vi "VI Tree.vi"   [LabVIEW 2012, in "Lake Shore Cryotronics 370.lvlib"]
doc: "This is the instrument driver for the LakeShore Cryotronics Model 370 AC Resistance Bridge. The VI Tree displays all the user-callable VIs of the instrument driver in an organized table."
uses:
  <instrlib>/Lake Shore Cryotronics 370/Lake Shore Cryotronics 370.lvlib
panel:
  # "(c) 2001- 2009 National Instruments.  ALL RIGHTS RESERVED."
  # "SEE DIAGRAM\nFOR VI TREE."
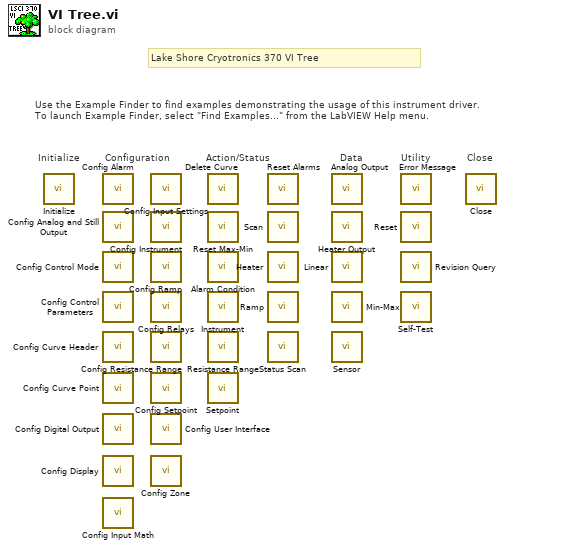
[diagram p0: block diagram]
diagram:
  # "Lake Shore Cryotronics 370 VI Tree"
  # "Initialize"
  # "Close"
  # "Action/Status"
  # "Data"
  # "Utility"
  # "Configuration"
  # "Use the Example Finder to find examples demonstrating the usage of this instrument driver.\nTo launch Example Finder, select \"Find Examples...\" from the LabVIEW Help menu."
  n1 = call <instrlib>:"Initialize.vi"() -> ()  [unwired: 14 in, 2 out]
  n2 = call <instrlib>:"Config Alarm.vi"() -> ()  [unwired: 14 in, 2 out]
  n3 = call <instrlib>:"Config Analog and Still Output.vi"() -> ()  [unwired: 14 in, 2 out]
  n4 = call <instrlib>:"Config Control Mode.vi"() -> ()  [unwired: 14 in, 2 out]
  n5 = call <instrlib>:"Config Control Parameters.vi"() -> ()  [unwired: 14 in, 2 out]
  n6 = call <instrlib>:"Config Curve Header.vi"() -> ()  [unwired: 14 in, 2 out]
  n7 = call <instrlib>:"Config Curve Point.vi"() -> ()  [unwired: 14 in, 2 out]
  n8 = call <instrlib>:"Config Digital Output.vi"() -> ()  [unwired: 14 in, 2 out]
  n9 = call <instrlib>:"Config Display.vi"() -> ()  [unwired: 14 in, 2 out]
  n10 = call <instrlib>:"Config Input Math.vi"() -> ()  [unwired: 26 in, 2 out]
  n11 = call <instrlib>:"Config Input Settings.vi"() -> ()  [unwired: 14 in, 2 out]
  n12 = call <instrlib>:"Config Instrument.vi"() -> ()  [unwired: 14 in, 2 out]
  n13 = call <instrlib>:"Config Ramp.vi"() -> ()  [unwired: 14 in, 2 out]
  n14 = call <instrlib>:"Config Relays.vi"() -> ()  [unwired: 14 in, 2 out]
  n15 = call <instrlib>:"Config Resistance Range.vi"() -> ()  [unwired: 14 in, 2 out]
  n16 = call <instrlib>:"Config Setpoint.vi"() -> ()  [unwired: 14 in, 2 out]
  n17 = call <instrlib>:"Config User Interface.vi"() -> ()  [unwired: 14 in, 2 out]
  n18 = call <instrlib>:"Config Zone.vi"() -> ()  [unwired: 26 in, 2 out]
  n19 = call <instrlib>:"Delete Curve.vi"() -> ()  [unwired: 14 in, 2 out]
  n20 = call <instrlib>:"Reset Max-Min.vi"() -> ()  [unwired: 14 in, 2 out]
  n21 = call <instrlib>:"Alarm Condition.vi"() -> ()  [unwired: 12 in, 4 out]
  n22 = call <instrlib>:"Instrument.vi"() -> ()  [unwired: 9 in, 7 out]
  n23 = call <instrlib>:"Resistance Range.vi"() -> ()  [unwired: 9 in, 7 out]
  n24 = call <instrlib>:"Setpoint.vi"() -> ()  [unwired: 13 in, 3 out]
  n25 = call <instrlib>:"Reset Alarms.vi"() -> ()  [unwired: 14 in, 2 out]
  n26 = call <instrlib>:"Scan.vi"() -> ()  [unwired: 14 in, 2 out]
  n27 = call <instrlib>:"Heater.vi"() -> ()  [unwired: 13 in, 3 out]
  n28 = call <instrlib>:"Ramp.vi"() -> ()  [unwired: 11 in, 5 out]
  n29 = call <instrlib>:"Status Scan.vi"() -> ()  [unwired: 12 in, 4 out]
  n30 = call <instrlib>:"Analog Output.vi"() -> ()  [unwired: 13 in, 3 out]
  n31 = call <instrlib>:"Heater Output.vi"() -> ()  [unwired: 13 in, 3 out]
  n32 = call <instrlib>:"Linear.vi"() -> ()  [unwired: 13 in, 3 out]
  n33 = call <instrlib>:"Min-Max.vi"() -> ()  [unwired: 12 in, 4 out]
  n34 = call <instrlib>:"Sensor.vi"() -> ()  [unwired: 11 in, 5 out]
  n35 = call <instrlib>:"Error Message.vi"() -> ()  [unwired: 11 in, 5 out]
  n36 = call <instrlib>:"Reset.vi"() -> ()  [unwired: 14 in, 2 out]
  n37 = call <instrlib>:"Revision Query.vi"() -> ()  [unwired: 10 in, 6 out]
  n38 = call <instrlib>:"Self-Test.vi"() -> ()  [unwired: 12 in, 4 out]
  n39 = call <instrlib>:"Close.vi"() -> ()  [unwired: 15 in, 1 out]
